vi "标样核查配置.vi"() -> (2 "确认输出":bool)   [LabVIEW 2016, in "斯坦道多参数.lvlib"]
uses:
  <vilib>/Utility/config.llb/NI_LVConfig.lvlib
panel:
  in  "保存组数":dbl=1.0
  in  "浊度启用":bool
  in  "电导率启用":bool
  in  "溶解氧启用":bool
  in  "pH启用":bool
  in  "浊度标样值":dbl caption="浊度"
  in  "电导率标样值":dbl caption="电导率"
  in  "溶解氧标样值":dbl caption="溶解氧"
  in  "pH标样值":dbl caption="pH"
  in  "取消":bool
  in  "确定":bool
  in  "数据保存间隔":dbl=1.0
  # "请输入数据保存间隔"
  # "保存组数"
  # "min"
  # "组"
  # "请选择启动项"
  # "请输入各参数标样值"
  # "mg/L"
  # "μS/cm"
  # "NTU"
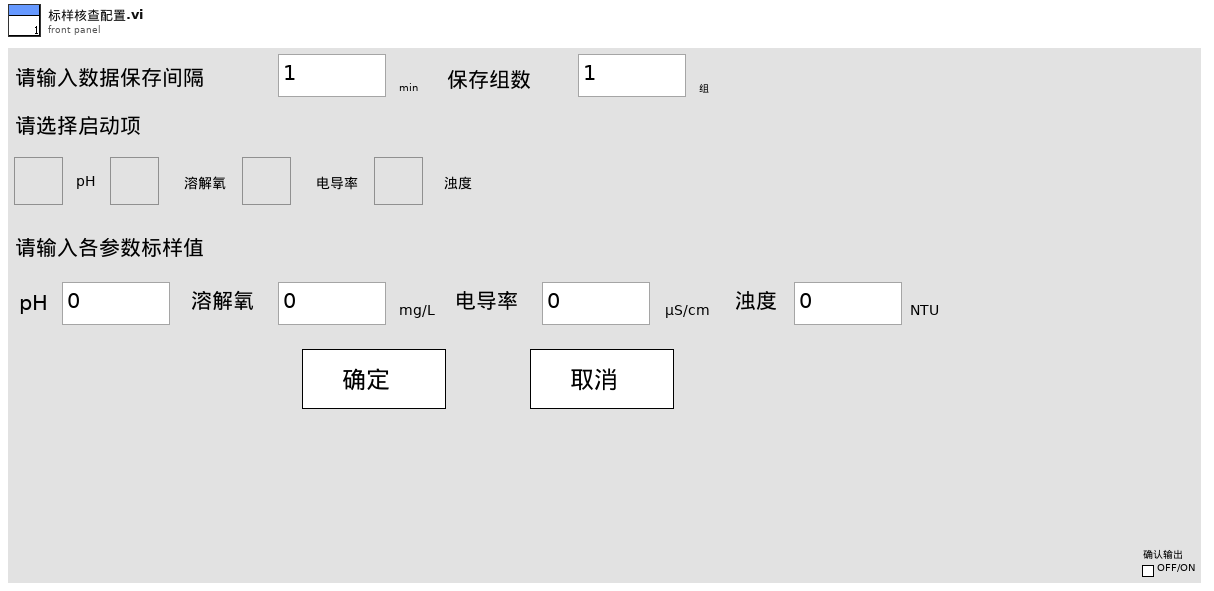
[diagram p1: front panel]
types:
  T1 = cluster{"数据保存间隔":dbl, "保存组数":dbl, "水温标样值":dbl, "pH标样值":dbl, "溶解氧标样值":dbl, "电导率标样值":dbl, "浊度标样值":dbl, "pH启用":bool, "溶解氧启用":bool, "电导率启用":bool, "浊度启用":bool}
  T2 = typedef "NI_LVConfig.lvlib/Config Data RefNum.ctl" = refnum<k1>
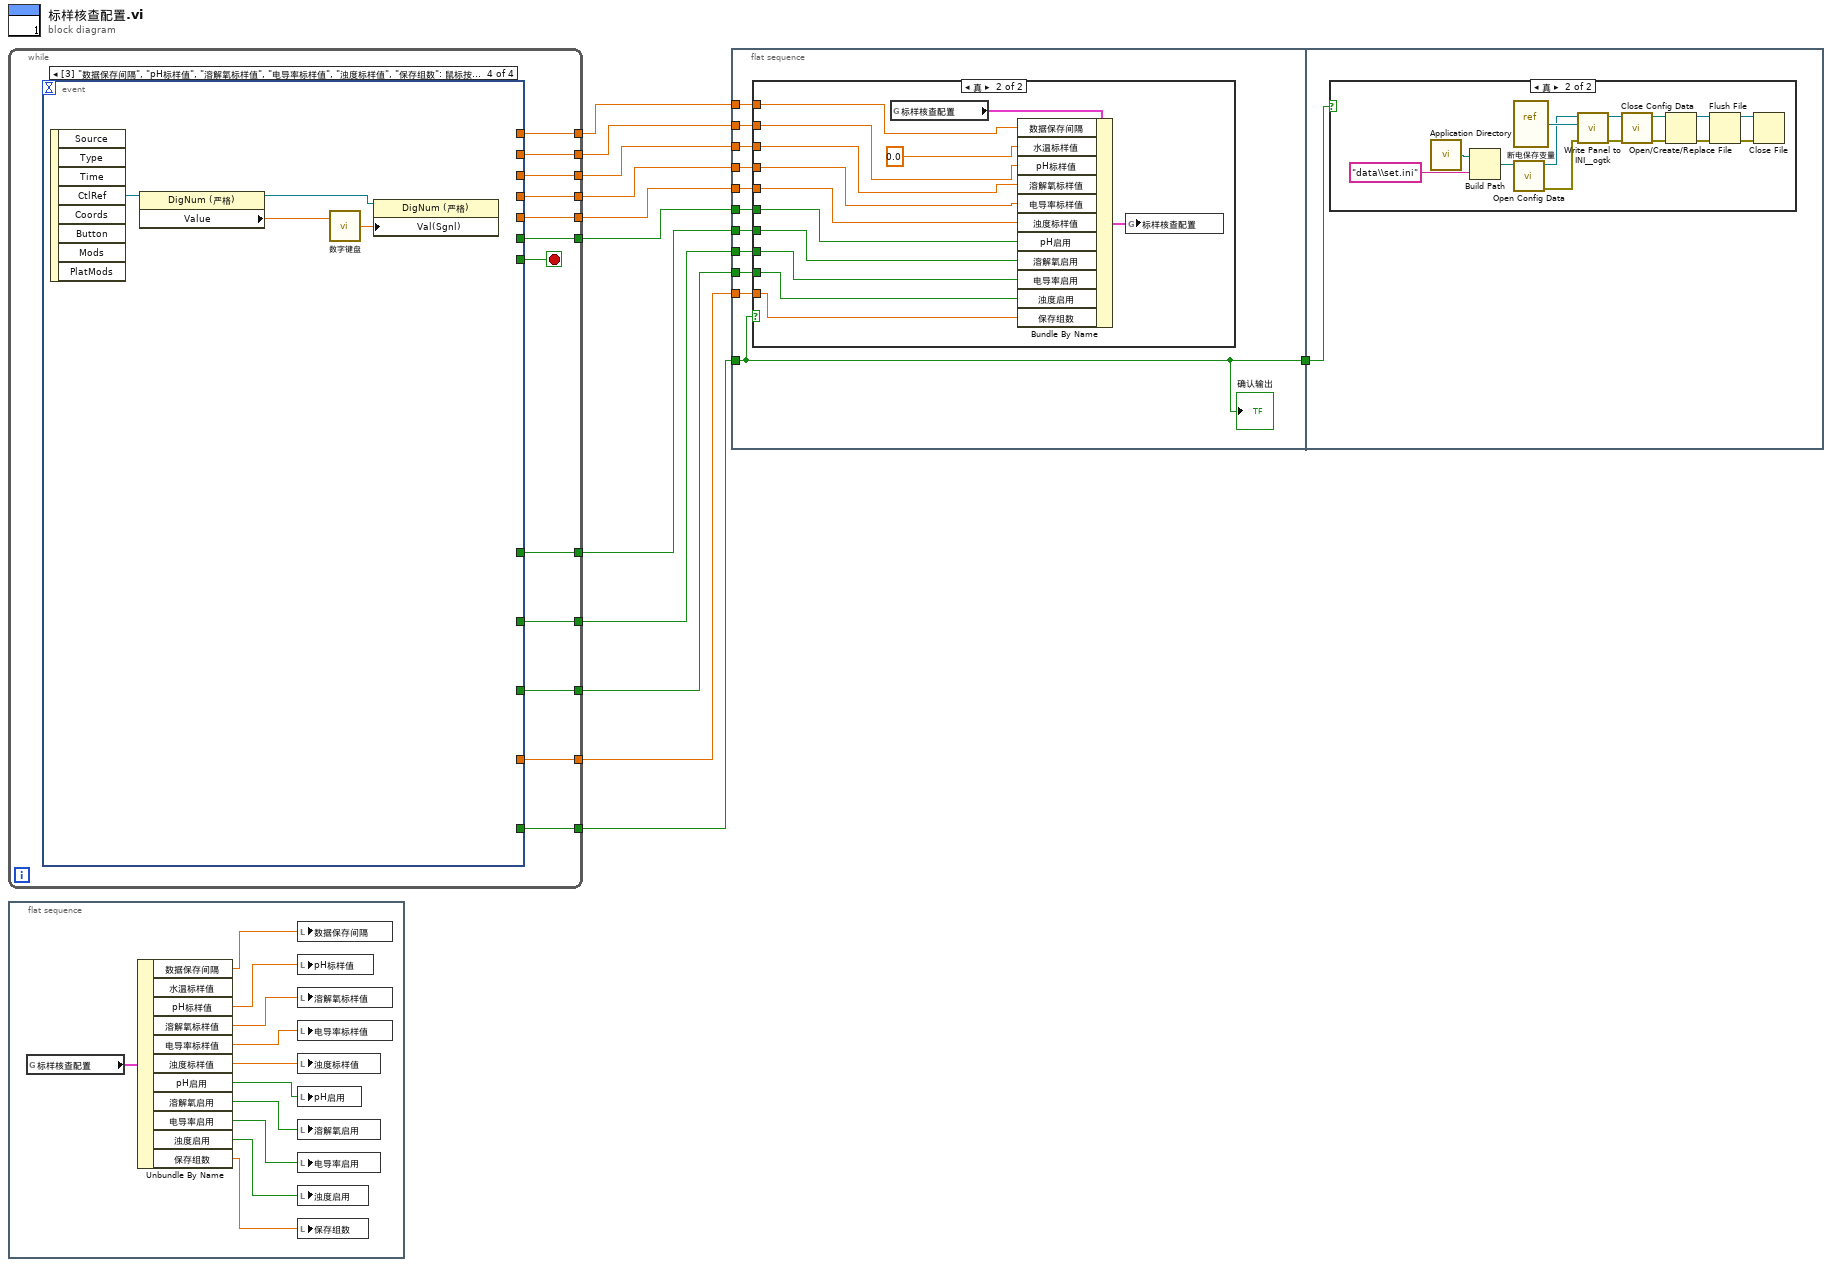
[diagram p0: block diagram]
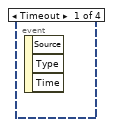
[diagram p4: hidden frame]
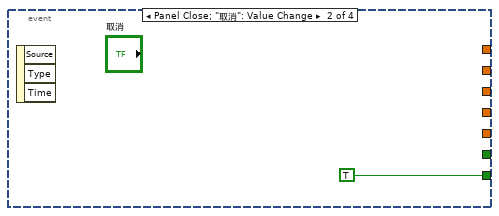
[diagram p5: hidden frame]
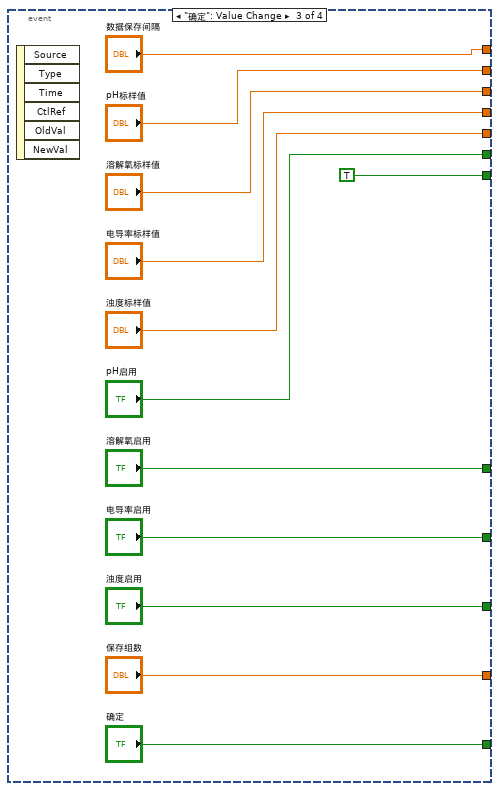
[diagram p6: hidden frame]
diagram:
  n1 = while {
    tunnel: [w23] -> w11
    tunnel: [w22] -> w12
    tunnel: [w21] -> w10
    tunnel: [w20] -> w9
    tunnel: [w19] -> w8
    tunnel: [w18] -> w7
    tunnel: [w17] -> w5
    tunnel: [w16] -> w4
    tunnel: [w15] -> w3
    tunnel: [w14] -> w2
    tunnel: [w13] -> w1
    stop <- w24 stop-if-true
    n2 = event shown="[3] \"数据保存间隔\", \"pH标样值\", \"溶解氧标样值\", \"电导率标样值\", \"浊度标样值\", \"保存组数\": 鼠标按下" {
      selector: _ -> [_ _ _ _]
      dyn-events: _ -> [_ _ _ _]
      timeout: _ -> [_ _ _ _]
      tunnel: [_ TRUE TRUE _] -> w24
      tunnel: [_ _ "数据保存间隔" _] -> w23
      tunnel: [_ _ "确定" _] -> w22
      tunnel: [_ _ "pH标样值" _] -> w21
      tunnel: [_ _ "溶解氧标样值" _] -> w20
      tunnel: [_ _ "电导率标样值" _] -> w19
      tunnel: [_ _ "浊度标样值" _] -> w18
      tunnel: [_ _ "浊度启用" _] -> w17
      tunnel: [_ _ "电导率启用" _] -> w16
      tunnel: [_ _ "pH启用" _] -> w15
      tunnel: [_ _ "溶解氧启用" _] -> w14
      tunnel: [_ _ "保存组数" _] -> w13
      event Timeout {
        n3 = event-data() -> ()  [unwired: 1 in, 3 out]
      }
      event Panel Close; "取消": Value Change {
        n4 = event-data() -> ()  [unwired: 1 in, 3 out]
      }
      event "确定": Value Change {
        n5 = event-data() -> ()  [unwired: 1 in, 6 out]
      }
      event "数据保存间隔", "pH标样值", "溶解氧标样值", "电导率标样值", "浊度标样值", "保存组数": Mouse Down {
        n6 = event-data() -> ("CtlRef"=w41:refnum<vi>)  [unwired: 1 in, 7 out]
        n7 = property class="DigNum (严格)"(reference=w41) -> (reference out=w38:refnum<vi>, "Value"=w40:dbl)  [unwired: 1 in, 1 out]
        n8 = call "数字键盘.vi"("OldNumber"=w40) -> ("NewNumber"=w39:dbl)  [unwired: 1 in]
        n9 = property class="DigNum (严格)"(reference=w38, "Val(Sgnl)"=w39) -> ()  [unwired: 1 in, 2 out]
      }
    }
  }
  n10 = flat-sequence {
    frame #0 {
      n11 = global read "断电保存变量.vi" "标样核查配置"() -> (w52:T1)
      n12 = Unbundle By Name(w52) -> ("数据保存间隔"=w51:dbl, "pH标样值"=w47:dbl, "溶解氧标样值"=w48:dbl, "电导率标样值"=w49:dbl, "浊度标样值"=w50:dbl, "pH启用"=w46:bool, "溶解氧启用"=w45:bool, "电导率启用"=w44:bool, "浊度启用"=w43:bool, "保存组数"=w42:dbl)  [unwired: 1 out]
      n13 = local write "数据保存间隔"(w51) -> ()
      n14 = local write "pH标样值"(w47) -> ()
      n15 = local write "溶解氧标样值"(w48) -> ()
      n16 = local write "电导率标样值"(w49) -> ()
      n17 = local write "浊度标样值"(w50) -> ()
      n18 = local write "pH启用"(w46) -> ()
      n19 = local write "溶解氧启用"(w45) -> ()
      n20 = local write "电导率启用"(w44) -> ()
      n21 = local write "浊度启用"(w43) -> ()
      n22 = local write "保存组数"(w42) -> ()
    }
  }
  n23 = flat-sequence {
    tunnel: w12 -> [w58]
    tunnel: w11 -> [w63]
    tunnel: w10 -> [w62]
    tunnel: w9 -> [w61]
    tunnel: w8 -> [w60]
    tunnel: w7 -> [w59]
    tunnel: [w58] -> w6
    tunnel: w5 -> [w57]
    tunnel: w4 -> [w56]
    tunnel: w3 -> [w55]
    tunnel: w2 -> [w54]
    tunnel: w1 -> [w53]
    tunnel: w6 -> [w77]
    frame #0 {
      n24 = case shown="真" w58 {
        tunnel: w63 -> [_ w76]
        tunnel: w62 -> [_ w75]
        tunnel: w61 -> [_ w74]
        tunnel: w60 -> [_ w73]
        tunnel: w59 -> [_ w72]
        tunnel: w57 -> [_ w70]
        tunnel: w56 -> [_ w69]
        tunnel: w55 -> [_ w68]
        tunnel: w54 -> [_ w67]
        tunnel: w53 -> [_ w64]
        frame False {
        }
        frame True {
          n25 = global read "断电保存变量.vi" "标样核查配置"() -> (w66:T1)
          n26 = Bundle By Name(cluster=w66, "数据保存间隔"=w76, "水温标样值"=0.0, "pH标样值"=w75, "溶解氧标样值"=w74, "电导率标样值"=w73, "浊度标样值"=w72, "pH启用"=w68, "溶解氧启用"=w67, "电导率启用"=w69, "浊度启用"=w70, "保存组数"=w64) -> (w65:T1)
          n27 = global write "断电保存变量.vi" "标样核查配置"(w65) -> ()
        }
      }
      "确认输出" <- w58
    }
    frame #1 {
      n28 = case shown="真" w77 {
        frame False {
        }
        frame True {
          n29 = call <vilib>:"Application Directory.vi"() -> ("Application Directory"=w82:path)
          n30 = Build Path(base path=w82, name or relative path="data\\set.ini" ("名称或相对路径")) -> (appended path=w83:path)
          n31 = vi-ref "断电保存变量.vi"() -> (w85:refnum<vi>)
          n32 = call <vilib>:"Open Config Data.vi"("configuration file path"=w83) -> ("error out"=w79:errorcluster, "refnum"=w78:T2)  [unwired: 8 in, 1 out]
          n33 = call <userlib>:"Write Panel to INI__ogtk.vi"("error in (no error)"=w79, "VI ref"=w85, "refnum"=w78) -> ("error out"=w81:errorcluster, "refnum out"=w80:T2)  [unwired: 7 in]
          n34 = call <vilib>:"Close Config Data.vi"("error in (no error)"=w81, "refnum"=w80) -> ("error out"=w89:errorcluster, "file path"=w88:path)  [unwired: 8 in]
          n35 = Open/Create/Replace File(file path (use dialog)=w88, error in=w89) -> (refnum out=w87:refnum<file>, error out=w86:errorcluster)  [unwired: 4 in, 1 out]
          n36 = Flush File(refnum=w87, error in=w86) -> (refnum out=w91:refnum<file>, error out=w90:errorcluster)
          n37 = Close File(refnum=w91, error in=w90) -> ()  [unwired: 2 out]
        }
      }
    }
  }
